vi "周围活着的元胞个数.vi"(9 "j":i32, 10 "i":i32, 11 "map输入":u8[][](array[numeric])) -> (2 "num":u8)   [LabVIEW 2015, in "生命游戏.lvlib" / "生命游戏.lvclass"]
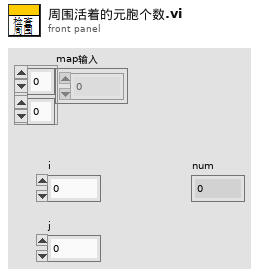
[diagram p1: front panel]
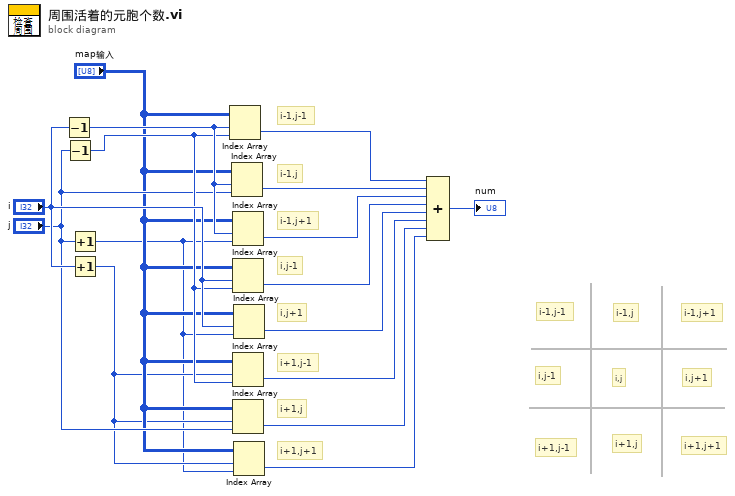
[diagram p0: block diagram]
diagram:
  # "i,j+1"
  # "i+1,j-1"
  # "i+1,j"
  # "i+1,j+1"
  # "i,j-1"
  # "i-1,j+1"
  # "i-1,j"
  # "i-1,j-1"
  # "i,j"
  # "i+1,j+1"
  # "i+1,j"
  # "i+1,j-1"
  # "i,j+1"
  # "i,j-1"
  # "i-1,j+1"
  # "i-1,j"
  # "i-1,j-1"
  n1 = Decrement(x="i") -> (x-1=w16:i32)
  n2 = Decrement(x="j") -> (x-1=w14:i32)
  n3 = Increment(x="j") -> (x+1=w10:i32)
  n4 = Increment(x="i") -> (x+1=w11:i32)
  n5 = Index Array(array="map输入", index (row)=w16, index (col)=w14) -> (element=w9:u8)
  n6 = Index Array(array="map输入", index (row)=w16, index (col)="j") -> (element=w8:u8)
  n7 = Index Array(array="map输入", index (row)=w16, index (col)=w10) -> (element=w7:u8)
  n8 = Index Array(array="map输入", index (row)="i", index (col)=w14) -> (element=w6:u8)
  n9 = Index Array(array="map输入", index (row)=w11, index (col)=w14) -> (element=w4:u8)
  n10 = Index Array(array="map输入", index (row)=w11, index (col)="j") -> (element=w3:u8)
  n11 = Index Array(array="map输入", index (row)="i", index (col)=w10) -> (element=w5:u8)
  n12 = Index Array(array="map输入", index (row)=w11, index (col)=w10) -> (element=w2:u8)
  n13 = Compound Arithmetic op=ADD(w9, w8, w7, w6, w5, w4, w3, w2) -> (→"num":u8)
